vi "_AbilityLog.vi"(11 "Log Entry":string) -> ()   [LabVIEW 2022 SP3, in "FlexBlocks Support.lvlib"]
uses:
  FlexBlocks Support.lvlib
panel:
  in  "Clear":bool
  out "String":string
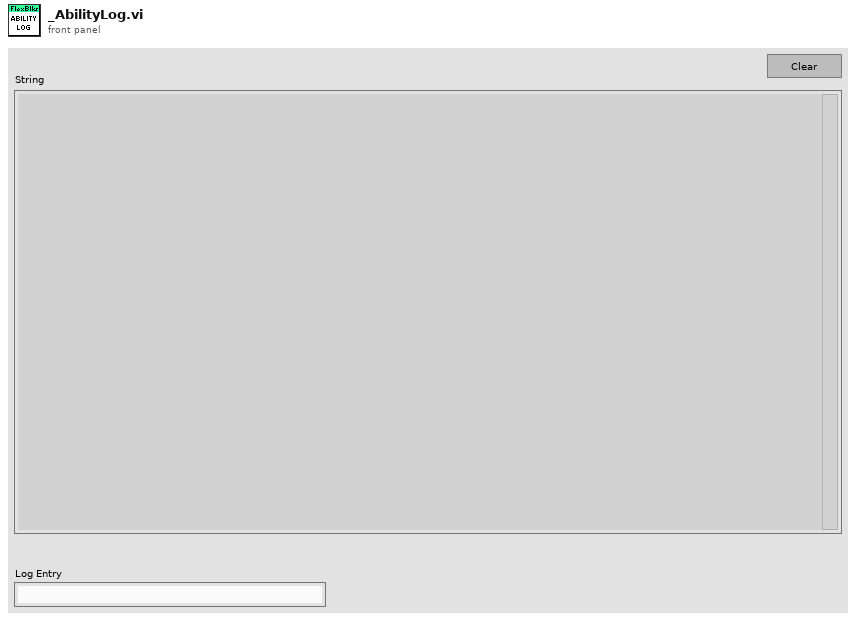
[diagram p1: front panel]
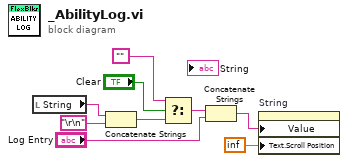
[diagram p0: block diagram]
diagram:
  n1 = local read "String"() -> (w9:string)
  n2 = Concatenate Strings(w9, "\r\n") -> (w6:string)
  n3 = Select(t="", s="Clear", f=w6) -> (s? t:f=w3:string)
  n4 = Concatenate Strings(w3, "Log Entry") -> (w1:string)
  n5 = property on="String" class="Str"("Value"=w1, "Text.Scroll Position"=inf) -> ()  [unwired: 2 in, 2 out]
